vi "Call Mock Transceiver Functions.vi"(6 "Fail to transmit?":bool, 8 "error in":errorcluster, 9 "transceiver settings":T1, 10 "Transfer Groups Configurations":T2[](array[typedef]) {"Transfers"."channel configurations"."buffer offset" format="%d bytes"}) -> (0 "error out":errorcluster, 2 "actual result":string)   [LabVIEW 2017, in "Transceiver Test Cases.lvclass"]
uses:
  Transceiver Test Cases.lvclass
  Configuration/Public/Controls/DSF Engine Transfer Group Configuration.ctl
  Configuration/Public/Controls/DSF Direction.ctl
  Configuration/Public/Controls/DSF Timing Info.ctl
  Configuration/Public/Controls/DSF Engine Transfer Configuration.ctl
  Configuration/Public/Controls/DSF Byte Order.ctl
  Configuration/Public/Controls/DSF Engine Channel Configuration.ctl
  Configuration/Public/Controls/DSF Data Type.ctl
  Configuration/Public/Controls/DSF Settings Info.ctl
  MockTransceiver.lvclass
  Engine/Classes/Transfer Group/Transfer Group.lvclass
  DSF Core.lvlib
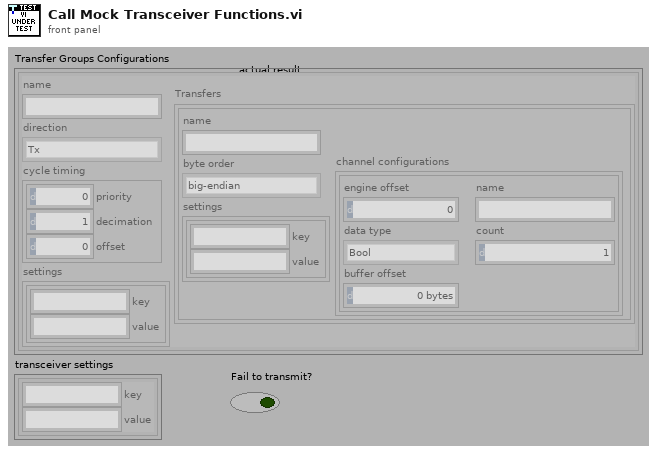
[diagram p1: front panel]
types:
  T1 = typedef "DSF Core.lvlib/DSF Settings Info.ctl" = cluster{"key":string, "value":string}[]
  T2 = typedef "DSF Core.lvlib/DSF Engine Transfer Group Configuration.ctl" = cluster{"name":string, "direction":T3, "cycle timing":T4, "Transfers":T5[], "settings":T1}
  T3 = typedef "DSF Core.lvlib/DSF Direction.ctl" = enum8{"Tx", "Rx"}
  T4 = typedef "DSF Core.lvlib/DSF Timing Info.ctl" = cluster{"priority":u64, "decimation":u64, "offset":u64}
  T5 = typedef "DSF Core.lvlib/DSF Engine Transfer Configuration.ctl" = cluster{"name":string, "byte order":T6, "channel configurations":T7[], "settings":T1}
  T6 = typedef "DSF Core.lvlib/DSF Byte Order.ctl" = enum8{"big-endian", "little-endian"}
  T7 = typedef "DSF Core.lvlib/DSF Engine Channel Configuration.ctl" = cluster{"engine offset":u64, "name":string, "data type":T8, "count":u64, "buffer offset":u64}
  T8 = typedef "DSF Core.lvlib/DSF Data Type.ctl" = enum8{"Bool", "SGL", "DBL", "I8", "I16", "I32", "I64", "U8", "U16", "U32", "U64"}
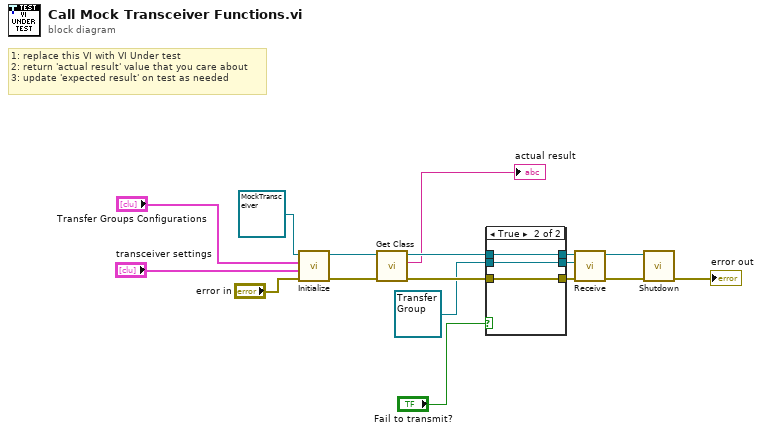
[diagram p0: block diagram]
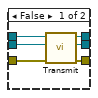
[diagram p2: hidden frame]
diagram:
  # "1: replace this VI with VI Under test\n2: return 'actual result' value that you care about\n3: update 'expected result' on test as needed"
  n1 = call-dynamic "Initialize.vi"("error in (no error)"="error in", "transceiver settings"="transceiver settings", "Transfer Groups Configurations"="Transfer Groups Configurations", "MockTransceiver in"=refnum<class "MockTransceiver.lvclass"> refnum) -> ("error out"=w17:errorcluster, "MockTransceiver out"=w16:refnum<class "MockTransceiver.lvclass">)  [unwired: 6 in]
  n2 = call-dynamic "Get Class.vi"("error in (no error)"=w17, "MockTransceiver in"=w16) -> ("error out"=w15:errorcluster, "class"=→"actual result":string, "MockTransceiver out"=w14:refnum<class "MockTransceiver.lvclass">)  [unwired: 7 in]
  n3 = case shown="True" "Fail to transmit?" {
    tunnel: w15 -> [w23 w24]
    tunnel: w14 -> [w22 w26]
    tunnel: [w21 w24] -> w13
    tunnel: [w20 w25] -> w12
    tunnel: [w19 w26] -> w11
    tunnel: refnum<class "Transfer Group.lvclass"> refnum ("Transfer Group in") -> [w18 w25]
    frame False {
      n4 = call-dynamic "Transmit.vi"("error in (no error)"=w23, "Transfer Group in"=w18, "MockTransceiver in"=w22) -> ("error out"=w21:errorcluster, "Transfer Group out"=w20:refnum<class "Transfer Group.lvclass">, "MockTransceiver out"=w19:refnum<class "MockTransceiver.lvclass">)  [unwired: 6 in]
    }
    frame True {
    }
  }
  n5 = call-dynamic "Receive.vi"("error in (no error)"=w13, "Transfer Group in"=w12, "MockTransceiver in"=w11) -> ("error out"=w10:errorcluster, "MockTransceiver out"=w9:refnum<class "MockTransceiver.lvclass">)  [unwired: 6 in, 1 out]
  n6 = call-dynamic "Shutdown.vi"("error in (no error)"=w10, "MockTransceiver in"=w9) -> ("error out"=→"error out":errorcluster)  [unwired: 8 in, 1 out]
